vi "Validate Instrument Revision.vi"(0 "VISA resource name":refnum<visa-resource-name>, 11 "error in (no error)":errorcluster) -> (4 "VISA resource name out":refnum<visa-resource-name>, 6 "Firmware Version":string, 10 "Model Number":string, 15 "error out":errorcluster)   [LabVIEW 2020, in "NH Research Regenerative Test Series.lvlib"]
doc: "Queries the instrument for the model number and firmware revision and validates them."
uses:
  Drivers-Essentials/NH Research Regenerative Test Series.lvlib
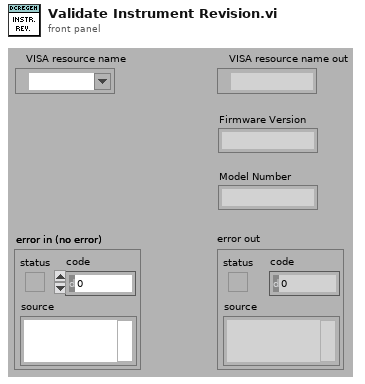
[diagram p1: front panel]
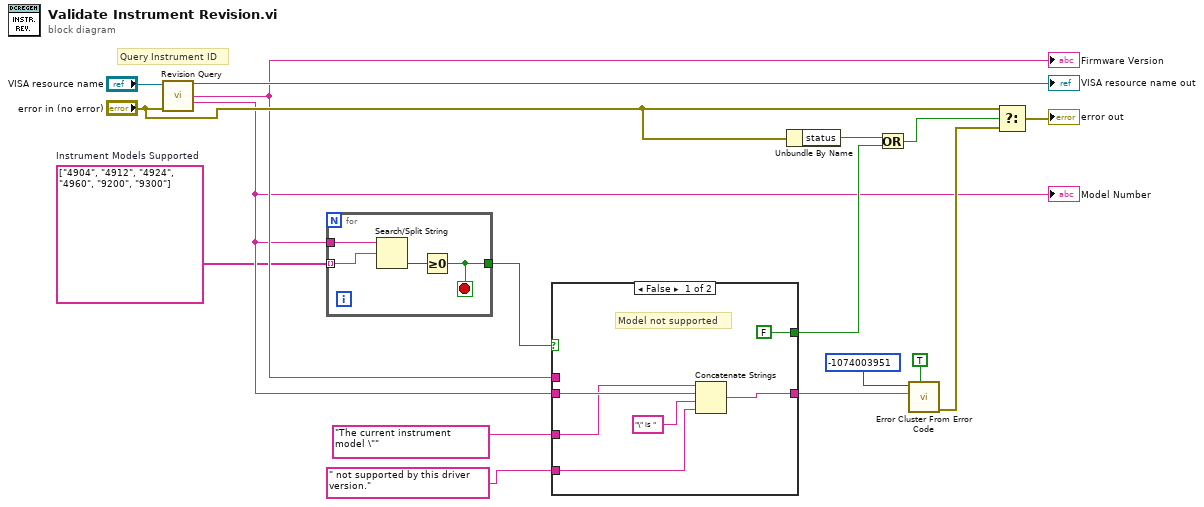
[diagram p0: block diagram]
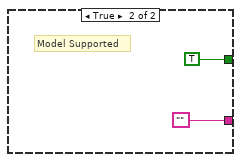
[diagram p2: hidden frame]
diagram:
  w2 = string[] ["4904", "4912", "4924", "4960", "9200", "9300"]  # Instrument Models Supported
  # "Query Instrument ID"
  n1 = call "Revision Query.vi"("VISA resource name"="VISA resource name", "error in (no error)"="error in (no error)") -> ("VISA resource name out"=→"VISA resource name out":refnum<visa-resource-name>, "Instrument Firmware Revision"=w4:string, "Instrument Model"=w3:string)  [unwired: 9 in, 2 out]
  "Firmware Version" <- w4
  "Model Number" <- w3
  n2 = for {
    tunnel: w3 -> [w21]
    tunnel: w2 -> [w20] mode=indexing
    tunnel: [w18] -> w1
    stop <- w18 stop-if-true
    n3 = Search/Split String(string=w21, search string/char (-)=w20) -> (offset of match=w19:i32)  [unwired: 1 in, 2 out]
    n4 = Greater Or Equal To 0?(x=w19) -> (x >= 0?=w18:bool)
  }
  n5 = case shown="False" w1 {
    tunnel: w3 -> [w26 _]
    tunnel: w4 -> [_ _]
    tunnel: "The current instrument model \"" ("Source (VI Name)") -> [w25 _]
    tunnel: " not supported by this driver version." ("Source (VI Name)") -> [w24 _]
    tunnel: [w23 ""] -> w9
    tunnel: [FALSE TRUE] -> w8
    frame False {
      # "Model not supported"
      n6 = Concatenate Strings(w25, w26, "\" is " ("string"), w24) -> (w23:string)
    }
    frame True {
      # "Model Supported"
    }
  }
  n7 = Unbundle By Name("error in (no error)") -> ("status"=w7:bool)
  n8 = Or(x=w7, y=w8) -> (x .or. y?=w6:bool)
  n9 = call "Error Cluster From Error Code.vi"("show call chain? (False)"=TRUE, "error message (\"\")"=w9, "error code (0)"=-1074003951 ("Code")) -> ("error out"=w15:errorcluster)  [unwired: 6 in]
  n10 = Select(t="error in (no error)", s=w6, f=w15) -> (s? t:f=→"error out":errorcluster)
